vi "xmlConfigRead.vi"(0 "path to XML document":path caption="XML文档路径", 1 "XPath expression":string caption="XPath表达式") -> (2 "OutParaVariant":variant, 3 "error out":errorcluster, 4 "OutParaArray":string[](array[string]))   [LabVIEW 2011]
doc: "加载类似如下这种结构的xml配置文件\n<?xml version=\"1.0\" encoding=\"UTF-8\"?>\n<ParameterList>\n <TerminationPoints>600</TerminationPoints>\n <ResultOffset>1</ResultOffset>\n <CableScale>9</CableScale>\n</ParameterList>\n得到一个变体，有三个属性，分别对应ParameterList的3个节点"
uses:
  <vilib>/xml/Load XML File.vi
  <vilib>/xml/NI_XML.lvlib
  program files/worksoftware/Labview/resource/objmgr/DOMUserDefRef.rc
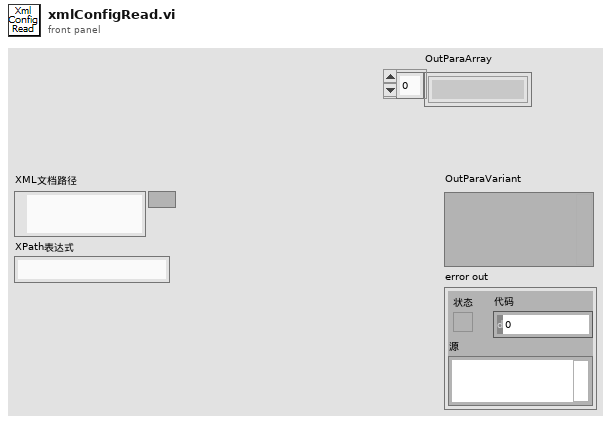
[diagram p1: front panel]
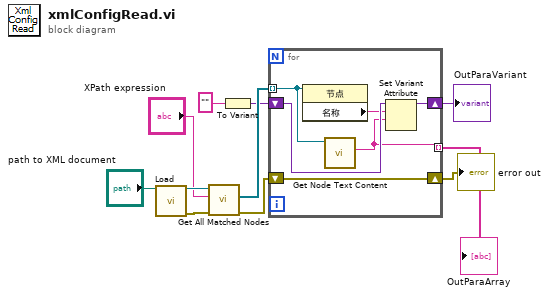
[diagram p0: block diagram]
diagram:
  n1 = call-poly <vilib>:"Load.vi"("path to XML document"="path to XML document") -> ("DOM document out"=w11:refnum<k20>, "error out"=w4:errorcluster)  [unwired: 12 in, 1 out]
  n2 = call <vilib>:"Get All Matched Nodes.vi"("error in (no error)"=w4, "XPath expression"="XPath expression", "node in"=w11) -> ("error out"=w3:errorcluster, "node result array"=w8:refnum<k20>[])  [unwired: 6 in, 1 out]
  n3 = To Variant(anything="") -> (Variant=w6:variant)
  n4 = for {
    tunnel: w8 -> [w17] mode=indexing
    shift-right: [w14] -> w5
    shift-left: w6 -> [w16]
    shift-right: [w13] -> w2
    shift-left: w3 -> [w13]
    tunnel: [w12] -> w1 mode=indexing
    n5 = property class="节点"(reference=w17) -> ("名称"=w15:string)  [unwired: 1 in, 2 out]
    n6 = call <vilib>:"Get Node Text Content.vi"("node in"=w17) -> ("node text"=w12:string)  [unwired: 8 in, 2 out]
    n7 = Set Variant Attribute(Variant=w16, name=w15, value=w12) -> (Variant out=w14:variant)  [unwired: 1 in, 2 out]
  }
  "OutParaVariant" <- w5
  "error out" <- w2
  "OutParaArray" <- w1
